vi "Draw Pie Chart.vi"(8 "error in (no error)":errorcluster, 11 "PieChart in":refnum<class "PieChart.lvclass">) -> (0 "error out":errorcluster, 3 "PieChart out":refnum<class "PieChart.lvclass">)   [LabVIEW 2018, in "PieChart.lvclass"]
uses:
  PieChart.lvclass
  <vilib>/picture/picture.llb/Draw True-Color Pixmap.vi
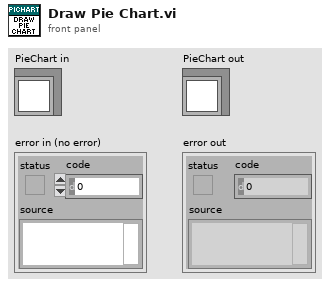
[diagram p1: front panel]
types:
  T1 = typedef "LVBoundsTypeDef.ctl" = cluster{"Width":u32, "Height":u32}
  T2 = typedef "PieChart.lvclass/State Data.ctl" = cluster{"Title":string, "Values[]":dbl[], "Labels[]":string[], "Colors[]":u32[], "Include Legend?":bool, "Include Title?":bool, "Title Font":T3, "Legend Font":T3, "Selection":i32, "Slice Positions":T4}
  T3 = typedef "LVFontTypeDef.ctl" = cluster{"Font Name":string, "Size":u16, "Bold":bool, "Italic":bool, "Underline":bool, "Strikeout":bool, "Color":u32}
  T4 = typedef "PieChart.lvclass/Pie info for Click.ctl" = cluster{"Slice Positions":cluster{"Start":i16, "End":i16}[], "Center Position":T1, "Radius":i16}
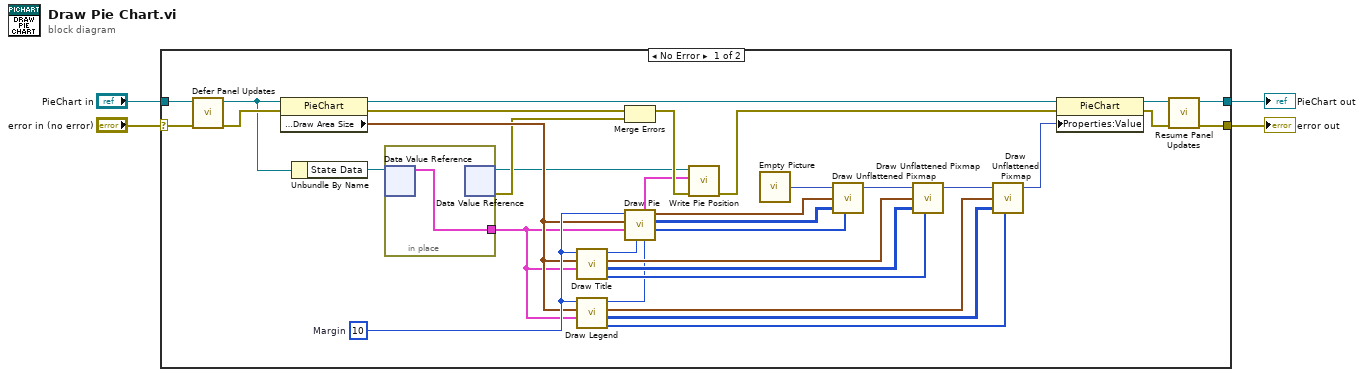
[diagram p0: block diagram]
diagram:
  n1 = case shown="No Error" "error in (no error)" {
    selector: "error in (no error)" -> [w9 w41]
    tunnel: [w5 w41] -> w3
    tunnel: [w7 w40] -> w1
    tunnel: "PieChart in" -> [w10 w40]
    frame No Error {
      w25 = i16 10  # Margin
      n2 = call "Defer Panel Updates.vi"("error in (no error)"=w9, "PieChart in"=w10) -> ("error out"=w38:errorcluster, "PieChart out"=w11:refnum<class "PieChart.lvclass">)  [unwired: 8 in]
      n3 = property class="PieChart"(reference=w11, error in=w38) -> (reference out=w16:refnum<class "PieChart.lvclass">, error out=w23:errorcluster, "Properties:Draw Area Size"=w24:T1)
      n4 = Unbundle By Name(w11) -> ("State Data"=w32:refnum<data-value>)
      n5 = in-place {
        in-place-border: [w39] -> w21
        n6 = in-place-dvr #1(w32) -> (w39:T2)  [unwired: 1 out]
        n7 = in-place-dvr #1() -> (w14:refnum<data-value>, w22:errorcluster)  [unwired: 1 in]
      }
      n8 = call "Draw Title.vi"("State Data"=w21, "Draw Area Size"=w24, "Margin"=w25) -> ("mask"=w20:u8[], "24-bit pixmap"=w29:u32[][], "Draw Position"=w30:cluster{"x":i16, "y":i16}, "Title Height"=w18:u32)  [unwired: 5 in]
      n9 = call "Draw Legend.vi"("State Data"=w21, "Properties:Draw Area Size"=w24, "Margin"=w25) -> ("mask"=w19:u8[], "24-bit pixmap"=w28:u32[][], "Draw Position"=w27:cluster{"x":i16, "y":i16}, "Legend Width"=w17:u32)  [unwired: 5 in]
      n10 = Merge Errors(w23, w22) -> (w15:errorcluster)
      n11 = call "Draw Pie.vi"("Legend Width"=w17, "Title Height"=w18, "State Data"=w21, "Draw Area Size in"=w24, "Margin"=w25) -> ("mask"=w26:u8[], "24-bit pixmap"=w33:u32[][], "Pie Draw Position"=w34:cluster{"Left":u32, "Top":u32}, "Pie info for Click"=w12:T4)  [unwired: 3 in]
      n12 = call "Write Pie Position.vi"("error in (no error)"=w15, "Slice Positions"=w12, "Data Value Reference in"=w14) -> ("error out"=w13:errorcluster)  [unwired: 8 in]
      n13 = call "Empty Picture"() -> ("empty picture"=w37:picture)
      n14 = call-poly <vilib>:"Draw Unflattened Pixmap.vi"("picture"=w37, "top left point(0, 0)"=w34, "data (RGB format)"=w33, "mask"=w26) -> ("new picture"=w35:picture)  [unwired: 5 in]
      n15 = call-poly <vilib>:"Draw Unflattened Pixmap.vi"("picture"=w35, "top left point(0, 0)"=w30, "data (RGB format)"=w29, "mask"=w20) -> ("new picture"=w31:picture)  [unwired: 5 in]
      n16 = call-poly <vilib>:"Draw Unflattened Pixmap.vi"("picture"=w31, "top left point(0, 0)"=w27, "data (RGB format)"=w28, "mask"=w19) -> ("new picture"=w36:picture)  [unwired: 5 in]
      n17 = property class="PieChart"(reference=w16, error in=w13, "Properties:Value"=w36) -> (reference out=w8:refnum<class "PieChart.lvclass">, error out=w6:errorcluster)
      n18 = call "Resume Panel Updates.vi"("error in (no error)"=w6, "PieChart in"=w8) -> ("error out"=w5:errorcluster, "PieChart out"=w7:refnum<class "PieChart.lvclass">)  [unwired: 8 in]
    }
    frame Error {
    }
  }
  "error out" <- w3
  "PieChart out" <- w1
